vi "rate_limiting.vi"(6 "Reset":bool, 7 "Parameters":T1={"Stimulus"={"Type"=enum."Off", "Phase"=0.0, "Amplitude"=[], "Injection point"=enum."Total pose", "Closed loop"=FALSE, "Offset"=[], "Tip -> world"=FALSE, "Frequency"=0.0, "Length"=0.0}, "Goal Filter A"={"Speedup max"=0.0, "Speedup thresh"=0.0, "Speedup nonlin"=0.0, "Filters"=[]}, "Mode controls"={"Hold"=FALSE, "Cancellation"=FALSE, "Goal filter"=FALSE, "Trigger"=FALSE}, "Manipulator type"=enum."Current piezo", "Manipulator calibration"={"Tool offsets"=[[0.0, 0.0, 36200.0]], "Handle light calibration"=[], "Base pivots"=[], "Output pivots"=[], "Length center"=0.0, "Workspace height"=[], "Workspace diameter"=[0.0, 0.0, 36200.0], "Stack travel"=400.0, "Saturation pos"=375.0, "Inverse filters"=[], "Strut length"=0.0}, "Network"={"Remote Host"="", "Send Status"=FALSE, "Send Port"=0, "Recv Commands"=FALSE, "Recv Port"=0}, "Goal Filter B"={"Speedup max"=0.0, "Speedup thresh"=0.0, "Speedup nonlin"=0.0, "Filters"=[]}, "Cancellation"={"KP"={"XY"=0.0, "Rxy"=0.0, "Z"=0.0, "Rz"=0.0}, "KI"=0.0, "KD"={"XY"=0.0, "Rxy"=0.0, "Z"=0.0, "Rz"=0.0}, "Max vel"=20.0, "Max acc"=0.001, "Int error limit"=3.0, "RCM gain"=0.0, "Bypass"=FALSE, "Degraded gain"=0.0}, "Transition time"=0.0, "Estimation"={"Link"={"Measure noise"=[], "Process noise"=[], "Alt process noise"=[], "Alt turnoff cycles"=20, "Innovation limit"=[], "Residue threshold"=0.0, "Enable"=FALSE}, "Handle"={"Measure noise"=[], "Process noise"=[], "State limits"=[], "Innovation limit"=[], "Prediction Lookahead"=0.0, "Enable"=FALSE}}} {"Transition time" format="%_3f"; "Cancellation"."Degraded gain" min=0 max=1 step=0.1 format="%#_3p"; "Cancellation"."RCM gain" min=0 max=1 step=0.1 format="%#_3p"; "Cancellation"."KD"."Rz" min=-1 max=1 step=0.01 format="%#_3p"; "Cancellation"."KD"."Rxy" min=-1 max=1 step=0.01 format="%#_3p"; "Cancellation"."KD"."Z" min=-1 max=1 step=0.01 format="%#_3p"; "Cancellation"."KD"."XY" min=-1 max=1 step=0.01 format="%#_3p"; "Cancellation"."KI" min=0 max=1 step=0.01 format="%#_3p"; "Cancellation"."KP"."Rz" min=-1 max=1 step=0.01 format="%#_3p"; "Cancellation"."KP"."Rxy" min=-1 max=1 step=0.01 format="%#_3p"; "Cancellation"."KP"."Z" min=-1 max=1 step=0.01 format="%#_3p"; "Cancellation"."KP"."XY" min=-1 max=1 step=0.01 format="%#_3p"; "Cancellation"."Max acc" format="%#_3p"; "Goal Filter B"."Filters"."V limit range" format="%_3p"; "Goal Filter B"."Filters"."V limit" format="%_3p"; "Goal Filter B"."Filters"."Upper Q" format="%_3f"; "Goal Filter B"."Filters"."Upper Fc" format="%_3p"; "Goal Filter B"."Filters"."Lower Q" format="%_3f"; "Goal Filter B"."Filters"."Scale factor" format="%_3f"; "Goal Filter B"."Filters"."Lower Fc" format="%_3p"; "Goal Filter B"."Speedup nonlin" format="%_3p"; "Goal Filter B"."Speedup thresh" format="%_3p"; "Goal Filter B"."Speedup max" format="%_3p"; "Manipulator calibration"."Strut length" format="%#_4p"; "Manipulator calibration"."Saturation pos" format="%#.1f"; "Manipulator calibration"."Stack travel" format="%#.1f"; "Manipulator calibration"."Length center" format="%#_4p"; "Manipulator calibration"."Output pivots" format="%#_6f"; "Manipulator calibration"."Base pivots" format="%#_6f"; "Manipulator calibration"."Handle light calibration" format="%#.1f"; "Goal Filter A"."Filters"."V limit range" format="%_3p"; "Goal Filter A"."Filters"."V limit" format="%_3p"; "Goal Filter A"."Filters"."Upper Q" format="%_3f"; "Goal Filter A"."Filters"."Upper Fc" format="%_3p"; "Goal Filter A"."Filters"."Lower Q" format="%_3f"; "Goal Filter A"."Filters"."Scale factor" format="%_3f"; "Goal Filter A"."Filters"."Lower Fc" format="%_3p"; "Goal Filter A"."Speedup nonlin" format="%_3p"; "Goal Filter A"."Speedup thresh" format="%_3p"; "Goal Filter A"."Speedup max" format="%_3p"; "Stimulus"."Length" min=0.0 max=100.0 step=100.0 format="%#_4p"; "Stimulus"."Frequency" min=0.0 step=100.0 format="%#_4g"; "Stimulus"."Offset" format="%#_3p"; "Stimulus"."Amplitude" format="%#_3p"; "Stimulus"."Phase" min=-180.0 max=360.0 step=100.0 format="%#.2f"}, 9 "Link goal":sgl[](array[numeric])) -> (2 "Substituted goal":sgl[](array[numeric]))   [LabVIEW 2014]
uses:
  testing/Micron params.ctl
  testing/stimulus.ctl
  testing/injection_point.ctl
  filtering/goal_loop_parms.ctl
  testing/mode_conrols.ctl
  testing/manipulator_cal.ctl
  asap/labview/testing/probe_calibration.ctl
  host/network_params.ctl
  sq_control_params.ctl
  decoupled_gain.ctl
  estimation_controls.ctl
panel:
  out "Goal velocity (um/cycle)":sgl[](array[numeric])
  # "Locals:"
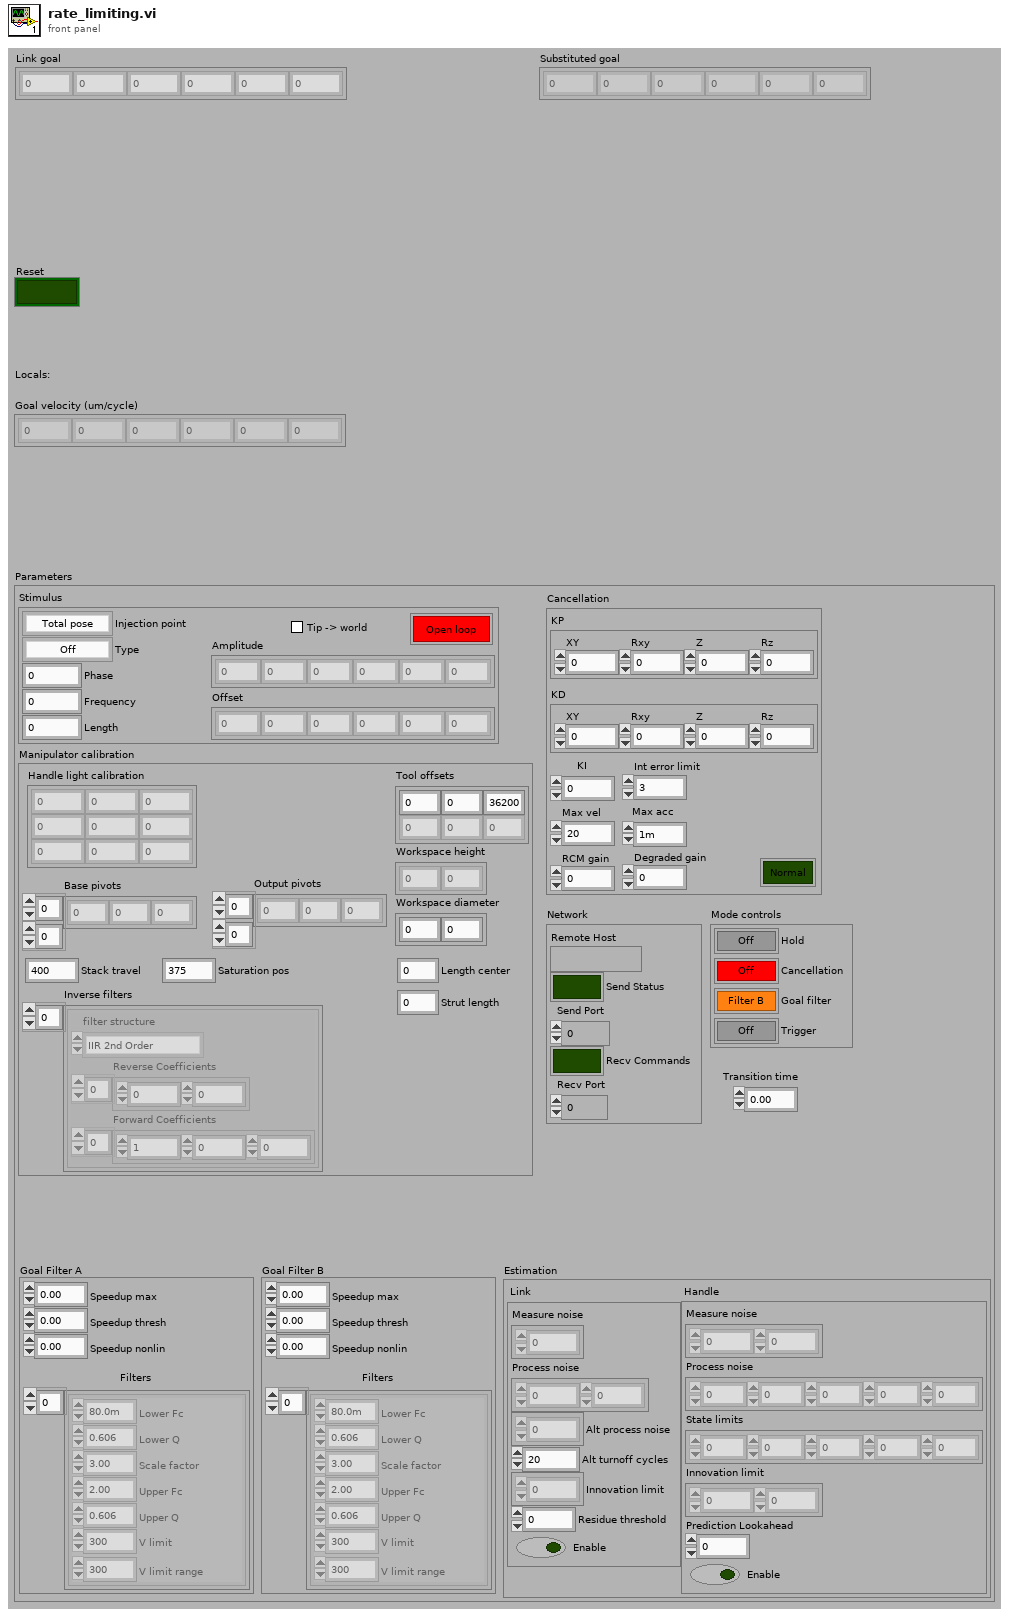
[diagram p1: front panel]
types:
  T1 = typedef "Micron params.ctl" = cluster{"Stimulus":T2, "Goal Filter A":T4, "Mode controls":T5, "Manipulator type":enum16{"Current piezo", "Voltage piezo"}, "Manipulator calibration":T6, "Network":T8, "Goal Filter B":T4, "Cancellation":T9, "Transition time":sgl, "Estimation":T11}
  T2 = typedef "stimulus.ctl" = cluster{"Type":enum16{"Off", "Step", "Sine", "Triangle", "Arbitrary"}, "Phase":dbl, "Amplitude":sgl[], "Injection point":T3, "Closed loop":bool, "Offset":sgl[], "Tip -> world":bool, "Frequency":dbl, "Length":dbl}
  T3 = typedef "injection_point.ctl" = enum16{"Total pose", "V limiter", "Goal ", "Link position", "KF link position", "Inverse kin", "Link goal", "Link error", "Controller", "Output", "Drive", "Light"}
  T4 = typedef "goal_loop_parms.ctl" = cluster{"Speedup max":sgl, "Speedup thresh":sgl, "Speedup nonlin":sgl, "Filters":cluster{"Lower Fc":sgl, "Lower Q":sgl, "Scale factor":sgl, "Upper Fc":sgl, "Upper Q":sgl, "V limit":sgl, "V limit range":sgl}[]}
  T5 = typedef "mode_conrols.ctl" = cluster{"Hold":bool, "Cancellation":bool, "Goal filter":bool, "Trigger":bool}
  T6 = typedef "manipulator_cal.ctl" = cluster{"Tool offsets":sgl[][], "Handle light calibration":T7, "Base pivots":sgl[][], "Output pivots":sgl[][], "Length center":sgl, "Workspace height":sgl[], "Workspace diameter":sgl[], "Stack travel":sgl, "Saturation pos":sgl, "Inverse filters":cluster{"filter structure":enum32{"IIR 2nd Order", "IIR 4th Order"}, "Reverse Coefficients":dbl[], "Forward Coefficients":dbl[]}[], "Strut length":sgl}
  T7 = typedef "probe_calibration.ctl" = sgl[][]
  T8 = typedef "network_params.ctl" = cluster{"Remote Host":string, "Send Status":bool, "Send Port":u16, "Recv Commands":bool, "Recv Port":u16}
  T9 = typedef "sq_control_params.ctl" = cluster{"KP":T10, "KI":sgl, "KD":T10, "Max vel":sgl, "Max acc":sgl, "Int error limit":sgl, "RCM gain":sgl, "Bypass":bool, "Degraded gain":sgl}
  T10 = typedef "decoupled_gain.ctl" = cluster{"XY":sgl, "Rxy":sgl, "Z":sgl, "Rz":sgl}
  T11 = typedef "estimation_controls.ctl" = cluster{"Link":cluster{"Measure noise":dbl[], "Process noise":dbl[], "Alt process noise":dbl[], "Alt turnoff cycles":i32, "Innovation limit":dbl[], "Residue threshold":dbl, "Enable":bool}, "Handle":cluster{"Measure noise":dbl[], "Process noise":dbl[], "State limits":dbl[], "Innovation limit":dbl[], "Prediction Lookahead":sgl, "Enable":bool}}
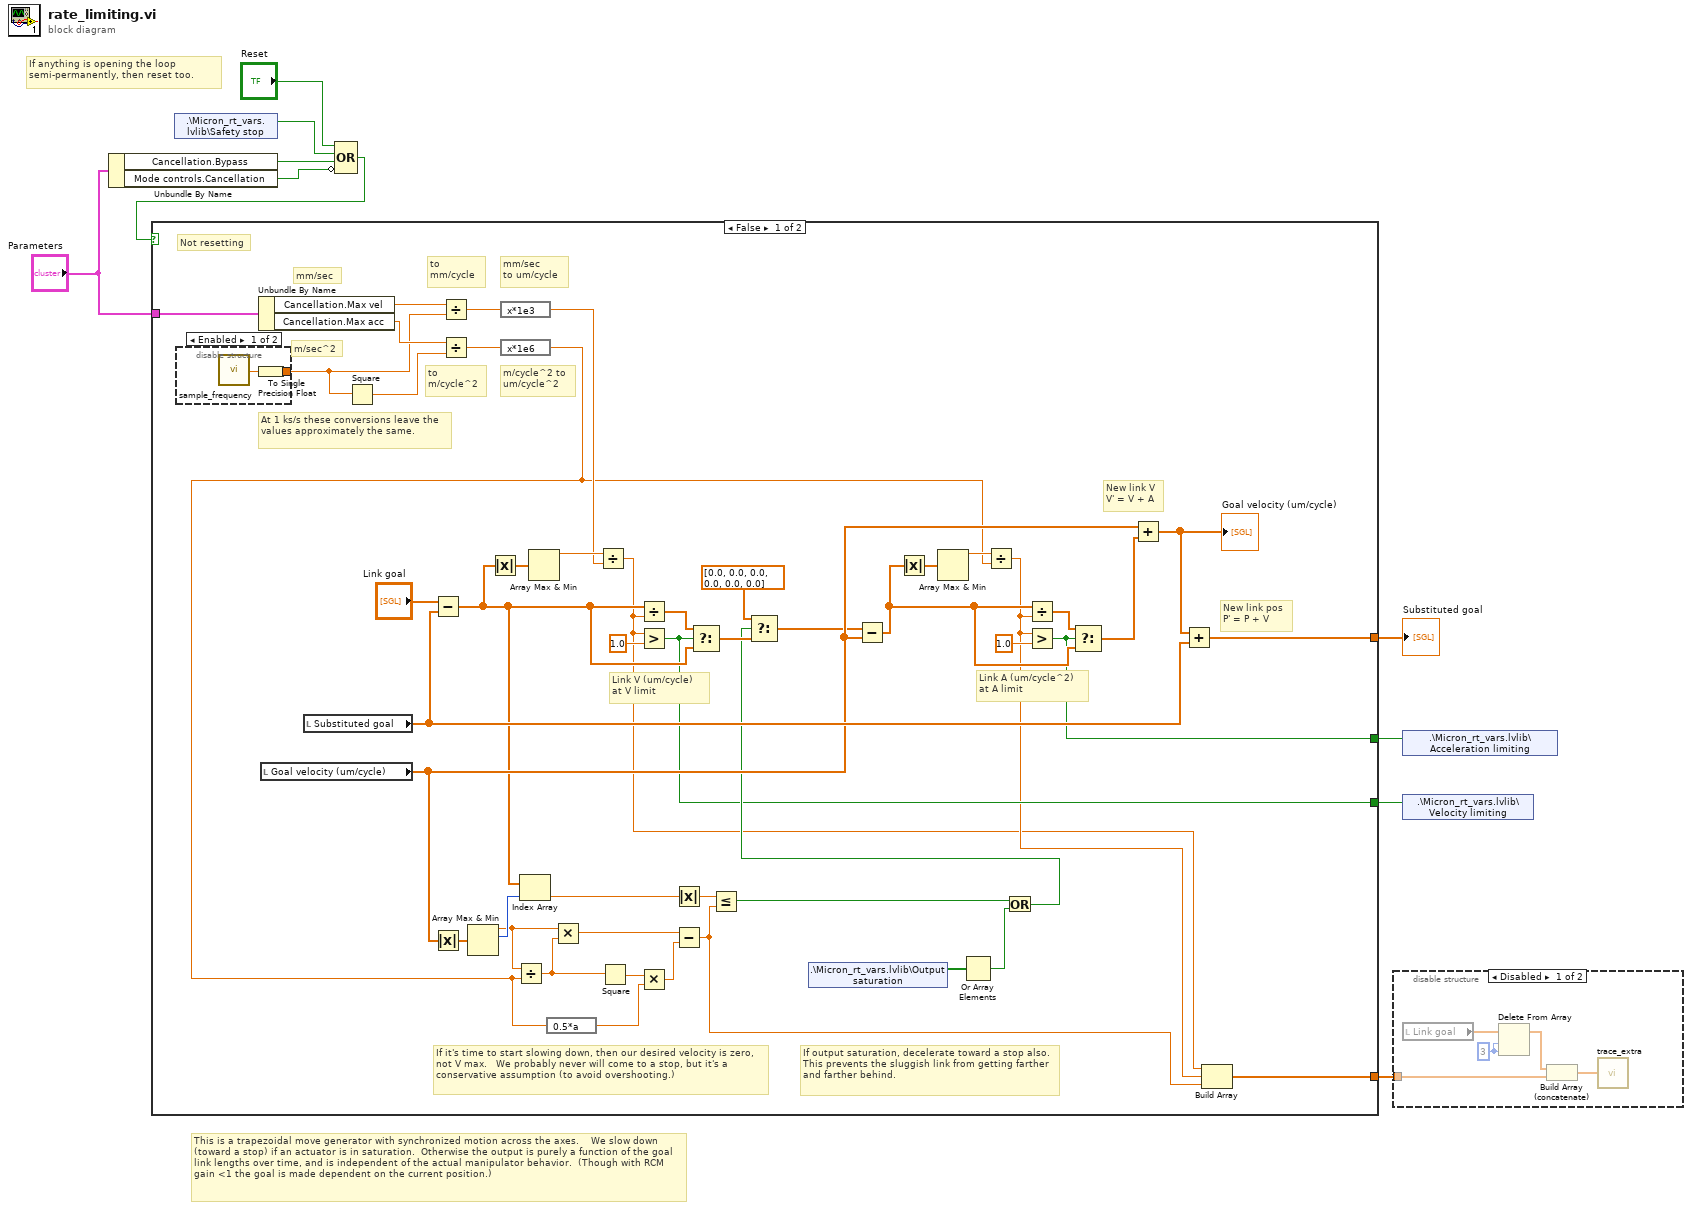
[diagram p0: block diagram]
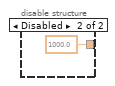
[diagram p3: hidden frame]
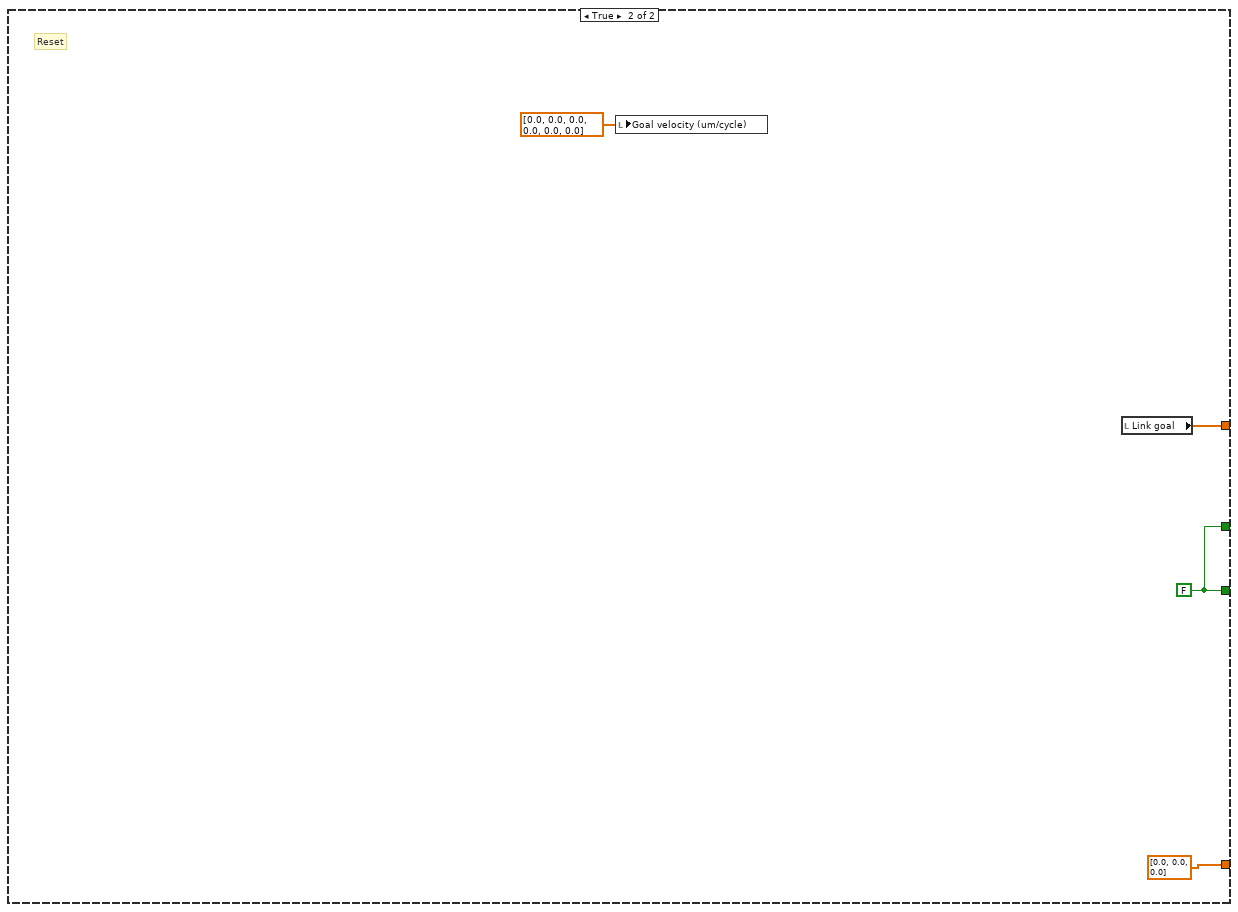
[diagram p4: hidden frame]
diagram:
  # "This is a trapezoidal move generator with synchronized motion across the axes.    We slow down (toward a stop) if an actuator is in saturation.  Otherwise the output is purely a function of the goal link lengths over time, and is independent of the actual manipulator behavior.  (Though with RCM gain <1 the goal is made dependent on the current position.)"
  # "If anything is opening the loop semi-permanently, then reset too."
  n1 = Unbundle By Name("Parameters") -> ("Cancellation.Bypass"=w9:bool, "Mode controls.Cancellation"=w6:bool)
  n2 = shared-variable ".\\Micron_rt_vars.lvlib\\Safety stop"() -> (w10:bool)  [unwired: 1 in, 1 out]
  n3 = Compound Arithmetic op=OR("Reset", w10, w9, invert w6) -> (w5:bool)
  n4 = case shown="False" w5 {
    tunnel: "Parameters" -> [w54 _]
    tunnel: [w43 w62] -> w4
    tunnel: [w35 sgl[] [0.0, 0.0, 0.0]] -> w3
    tunnel: [w16 w63] -> w2
    tunnel: [w15 w63] -> w1
    frame False {
      # "If output saturation, decelerate toward a stop also.  This prevents the sluggish link from getting farther and farther behind."
      # "If it's time to start slowing down, then our desired velocity is zero, not V max.   We probably never will come to a stop, but it's a conservative assumption (to avoid overshooting.)"
      # "New link pos\nP' = P + V"
      # "New link V\nV' = V + A"
      # "Link A (um/cycle^2)\nat A limit"
      # "Link V (um/cycle) \nat V limit"
      # "Not resetting"
      # "At 1 ks/s these conversions leave the values approximately the same."
      # "to \nm/cycle^2"
      # "m/sec^2"
      # "mm/sec"
      # "to\nmm/cycle"
      # "m/cycle^2 to\num/cycle^2"
      # "mm/sec \nto um/cycle"
      n5 = disable-structure shown="Enabled" {
        disable-tunnel: [w59 sgl 1000.0] -> w49
        frame Enabled {
          n6 = call "sample_frequency.vi"() -> ("Sample frequency"=w60:dbl)
          n7 = To Single Precision Float(number=w60) -> (single precision float=w59:sgl)
        }
        frame Disabled {
        }
      }
      n8 = Unbundle By Name(w54) -> ("Cancellation.Max vel"=w53:sgl, "Cancellation.Max acc"=w52:sgl)
      n9 = local read "Goal velocity (um/cycle)"() -> (w27:sgl[])
      n10 = local read "Substituted goal"() -> (w44:sgl[])
      n11 = Square(x=w49) -> (x^2=w50:sgl)
      n12 = Subtract(x="Link goal", y=w44) -> (x-y=w25:sgl[])
      n13 = Absolute Value(x=w27) -> (abs(x)=w34:sgl[])
      n14 = Divide(x=w53, y=w49) -> (x/y=w57:sgl)
      n15 = Divide(x=w52, y=w50) -> (x/y=w51:sgl)
      n16 = Array Max & Min(array=w34) -> (max value=w33:sgl, max index (indices)=w58:i32)  [unwired: 2 out]
      n17 = Absolute Value(x=w25) -> (abs(x)=w56:sgl[])
      n18 = expression code="x*1e3"(w57) -> (w48:sgl)
      n19 = expression code="x*1e6"(w51) -> (w26:sgl)
      n20 = Divide(x=w33, y=w26) -> (x/y=w32:sgl)
      n21 = Index Array(array=w25, index=w58) -> (element=w12:sgl)
      n22 = Array Max & Min(array=w56) -> (max value=w55:sgl)  [unwired: 3 out]
      n23 = expression code="0.5*a"(w26) -> (w30:sgl)
      n24 = Multiply(x=w33, y=w32) -> (x*y=w29:sgl)
      n25 = Divide(x=w55, y=w48) -> (x/y=w13:sgl)
      n26 = Square(x=w32) -> (x^2=w31:sgl)
      n27 = Divide(x=w25, y=w13) -> (x/y=w46:sgl[])
      n28 = Greater?(x=w13, y=sgl 1.0) -> (0:w15:bool)
      n29 = Multiply(x=w31, y=w30) -> (x*y=w28:sgl)
      n30 = Absolute Value(x=w12) -> (abs(x)=w11:sgl)
      n31 = Subtract(x=w29, y=w28) -> (x-y=w21:sgl)
      n32 = Select(t=w46, s=w15, f=w25) -> (s? t:f=w24:sgl[])
      n33 = Less Or Equal?(x=w11, y=w21) -> (x <= y?=w19:bool)
      n34 = shared-variable ".\\Micron_rt_vars.lvlib\\Output saturation"() -> (w20:bool[])  [unwired: 1 in, 1 out]
      n35 = Or Array Elements(Boolean array=w20) -> (logical OR=w17:bool)
      n36 = Or(x=w19, y=w17) -> (x .or. y?=w18:bool)
      n37 = Select(t=sgl[] [0.0, 0.0, 0.0, 0.0, 0.0, 0.0] ("Goal velocity (um/cycle)"), s=w18, f=w24) -> (s? t:f=w22:sgl[])
      n38 = Subtract(x=w22, y=w27) -> (x-y=w36:sgl[])
      n39 = Absolute Value(x=w36) -> (abs(x)=w42:sgl[])
      n40 = Array Max & Min(array=w42) -> (max value=w41:sgl)  [unwired: 3 out]
      n41 = Divide(x=w41, y=w26) -> (x/y=w14:sgl)
      n42 = Divide(x=w36, y=w14) -> (x/y=w39:sgl[])
      n43 = Greater?(x=w14, y=sgl 1.0) -> (0:w16:bool)
      n44 = Select(t=w39, s=w16, f=w36) -> (s? t:f=w38:sgl[])
      n45 = Add(x=w27, y=w38) -> (x+y=w37:sgl[])
      "Goal velocity (um/cycle)" <- w37
      n46 = Add(x=w37, y=w44) -> (x+y=w43:sgl[])
      n47 = Build Array(w13, w14, w21) -> (w35:sgl[])
    }
    frame True {
      w63 = FALSE
      # "Reset"
      n48 = local write "Goal velocity (um/cycle)"(sgl[] [0.0, 0.0, 0.0, 0.0, 0.0, 0.0] ("Goal velocity (um/cycle)")) -> ()
      n49 = local read "Link goal"() -> (w62:sgl[])
    }
  }
  "Substituted goal" <- w4
  n50 = disable-structure shown="Disabled" {
    disable-tunnel: w3 -> [w66 _]
    frame Disabled {
      w69 = 3 ("index")
      n51 = local read "Link goal"() -> (w70:sgl[])
      n52 = Delete From Array(array=w70, length=w69, index=w69) -> (array with subset deleted=w68:sgl[])  [unwired: 1 out]
      n53 = Build Array (concatenate)(w68, w66) -> (w67:sgl[])
      n54 = call "trace_extra.vi"("Extra trace data"=w67) -> ()  [unwired: 1 in]
    }
    frame Enabled {
    }
  }
  n55 = shared-variable ".\\Micron_rt_vars.lvlib\\Acceleration limiting"(w2) -> ()  [unwired: 2 out]
  n56 = shared-variable ".\\Micron_rt_vars.lvlib\\Velocity limiting"(w1) -> ()  [unwired: 2 out]
